vi "Iterator.vi"(8 "Final Value":dbl, 9 "Initial Value":dbl, 10 "Step":dbl, 11 "i":i32) -> (2 "End Loop":bool, 3 "Current Value":dbl)   [LabVIEW 2018]
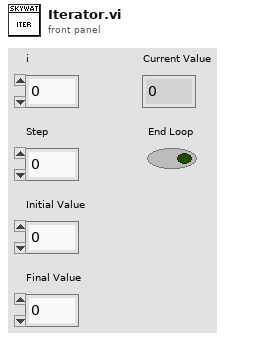
[diagram p1: front panel]
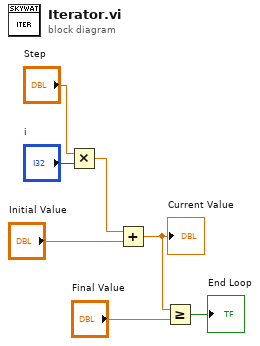
[diagram p0: block diagram]
diagram:
  n1 = Multiply(x="Step", y="i") -> (x*y=w3:dbl)
  n2 = Add(x=w3, y="Initial Value") -> (x+y=w7:dbl)
  "Current Value" <- w7
  n3 = Greater Or Equal?(x=w7, y="Final Value") -> (x >= y?=→"End Loop":bool)
